vi "Get System Name.vi"(8 "error in (no error)":errorcluster, 11 "Operator in":refnum<class "Operator.lvclass">) -> (0 "error out":errorcluster, 2 "System Name":string, 3 "Operator out":refnum<class "Operator.lvclass">)   [LabVIEW 2014, in "Operator.lvlib" / "Operator.lvclass"]
uses:
  Operator.lvclass
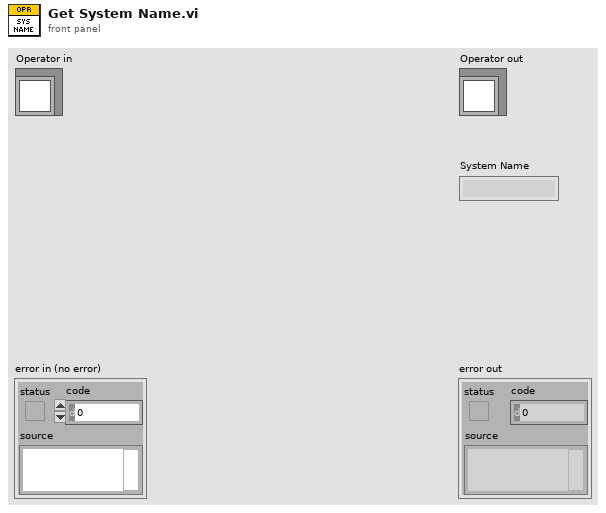
[diagram p1: front panel]
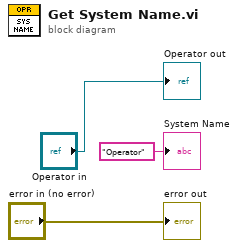
[diagram p0: block diagram]
diagram:
  "error out" <- "error in (no error)"
  "Operator out" <- "Operator in"
  "System Name" <- "Operator" ("System Name")
